vi "Return Transfer Group.vi"(8 "error in (no error)":errorcluster, 10 "Transfer Group in":refnum<class "Transfer Group.lvclass">, 11 "Transceiver Thread in":refnum<class "Plugin Thread.lvclass">) -> (0 "error out":errorcluster, 3 "Transceiver Thread out":refnum<class "Plugin Thread.lvclass">)   [LabVIEW 2020, in "DSF Core.lvlib" / "Plugin Thread.lvclass"]
uses:
  Thread/Plugin/Plugin Thread.lvclass
  Transfer Group/Transfer Group.lvclass
  Transfer Group/Transfer Group.lvclass/Transfer Group.ctl
  Timing/Timing.lvclass/Timing.ctl
  Thread/Plugin/Plugin Thread.lvclass/Plugin Thread.ctl
  Timing/Get Iteration.vi
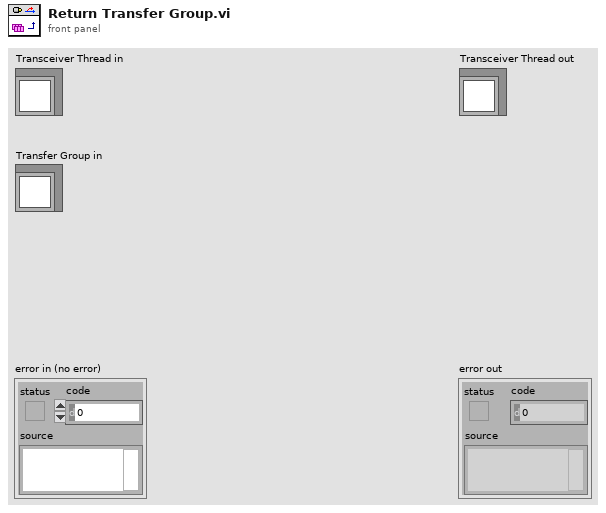
[diagram p1: front panel]
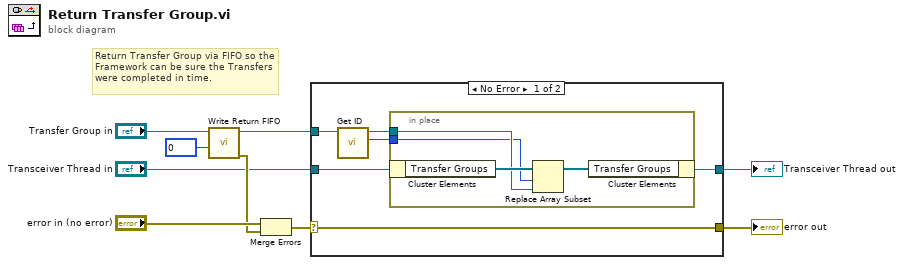
[diagram p0: block diagram]
diagram:
  # "Return Transfer Group via FIFO so the Framework can be sure the Transfers were completed in time."
  n1 = call "Write Return FIFO.vi"("timeout in ms (0)"=0, "Transfer Group in"="Transfer Group in") -> ("error out"=w6:errorcluster, "Transfer Group out"=w3:refnum<class "Transfer Group.lvclass">)  [unwired: 7 in, 1 out]
  n2 = Merge Errors("error in (no error)", w6) -> (w2:errorcluster)
  n3 = case shown="No Error" w2 {
    selector: w2 -> [w10 w21]
    tunnel: "Transceiver Thread in" -> [w15 w20]
    tunnel: [w12 w20] -> w4
    tunnel: w3 -> [w11 _]
    tunnel: [w10 w21] -> w1
    frame No Error {
      n4 = call "Get ID.vi"("Transfer Group in"=w11) -> ("id"=w13:i32, "Transfer Group out"=w14:refnum<class "Transfer Group.lvclass">)  [unwired: 9 in]
      n5 = in-place {
        in-place-border: w14 -> [w18]
        in-place-border: w13 -> [w17]
        n6 = in-place-cluster #1(w15) -> ("Transfer Groups"=w19:refnum<class "Transfer Group.lvclass">[])
        n7 = Replace Array Subset(array=w19, new element=w18, index=w17) -> (w16:refnum<class "Transfer Group.lvclass">[])
        n8 = in-place-cluster #1("Transfer Groups"=w16) -> (w12:refnum<class "Plugin Thread.lvclass">)
      }
    }
    frame Error {
    }
  }
  "error out" <- w1
  "Transceiver Thread out" <- w4
